vi "Add Noise.vi"(11 "Image In":u8[](array[numeric])) -> (3 "Image Out":u8[](array[numeric]))   [LabVIEW 2020]
uses:
  <vilib>/ptbypt/NI_PtbyPt.lvlib
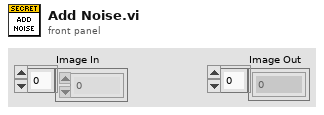
[diagram p1: front panel]
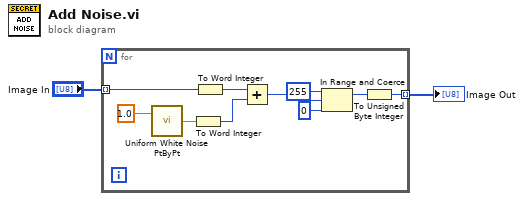
[diagram p0: block diagram]
diagram:
  n1 = for {
    tunnel: "Image In" -> [w12] mode=indexing
    tunnel: [w5] -> w1 mode=indexing
    n2 = call <vilib>:"Uniform White Noise PtByPt.vi"("amplitude"=1.0) -> ("uniform white noise"=w3:dbl)  [unwired: 2 in]
    n3 = To Word Integer(number=w3) -> (16bit integer=w10:i16)
    n4 = To Word Integer(number=w12) -> (16bit integer=w11:i16)
    n5 = Add(x=w11, y=w10) -> (x+y=w9:i16)
    n6 = In Range and Coerce(upper limit=i16 255, x=w9, lower limit=i16 0) -> (coerced(x)=w6:i16)  [unwired: 1 out]
    n7 = To Unsigned Byte Integer(number=w6) -> (unsigned 8bit integer=w5:u8)
  }
  "Image Out" <- w1
